vi "NanonisProperties_tessttttt.vi"(0 "Application reference":refnum<vi>, 5 "Ring":u16(ring) items=["all", "setpoint", "zread", "current", "frame", "follow me"], 11 "Error in":errorcluster, 12 "Z Write?":bool) -> (4 "Application ref out":refnum<vi>, 14 "tick count":u32, 15 "error out":errorcluster)   [LabVIEW 2019]
uses:
  <userlib>/Nanonis Prog Interface V5/Nanonis Prog Interface.lvlib
panel:
  out "Z Read (m)":sgl format="%#_6p"
  in  "Z Write (m)":sgl format="%#_6p"
  out "Setpoint (A)":sgl format="%#_6p"
  out "Current (pA)":sgl format="%#_6p"
  in  "Z pen (nm)":dbl
  in  "X pen (nm)":dbl
  out "Frame Size (m)":cluster{"Width":sgl, "Height":sgl} {"Height" format="%.2p"; "Width" format="%.2p"}
  out "Frame Origin (m)":cluster{"Xc":sgl, "Yc":sgl} {"Yc" format="%.2p"; "Xc" format="%.2p"}
  out "prog int?":bool
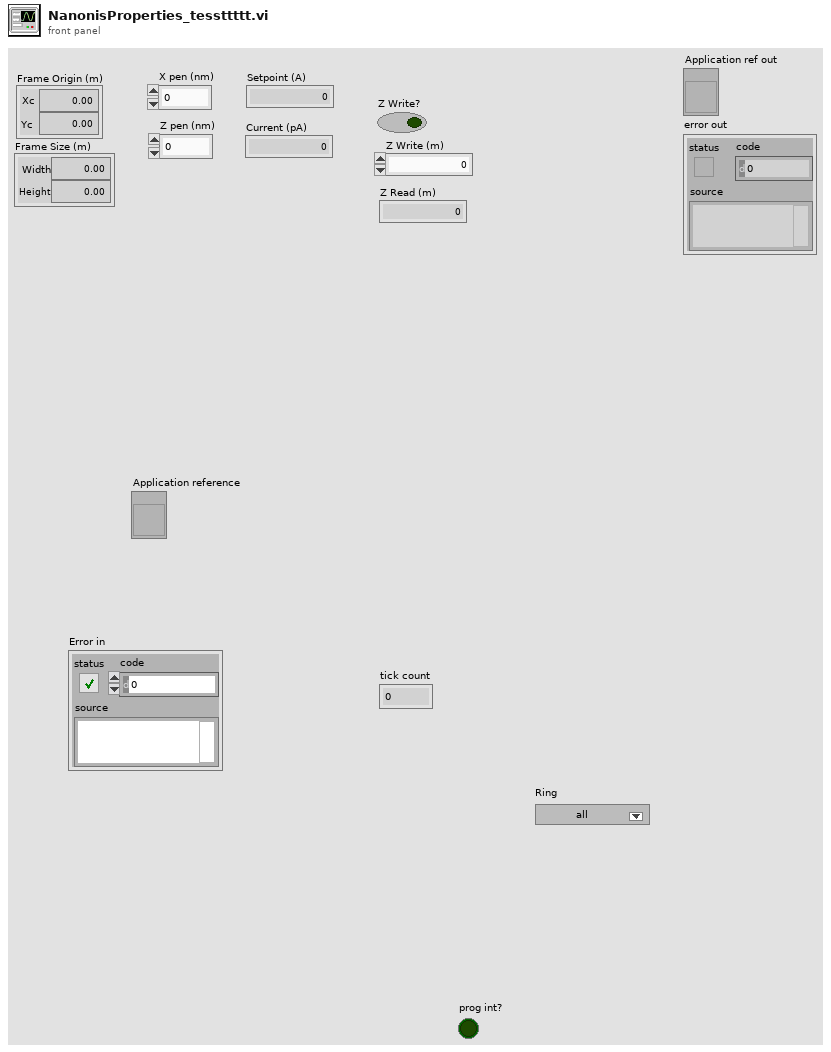
[diagram p1: front panel]
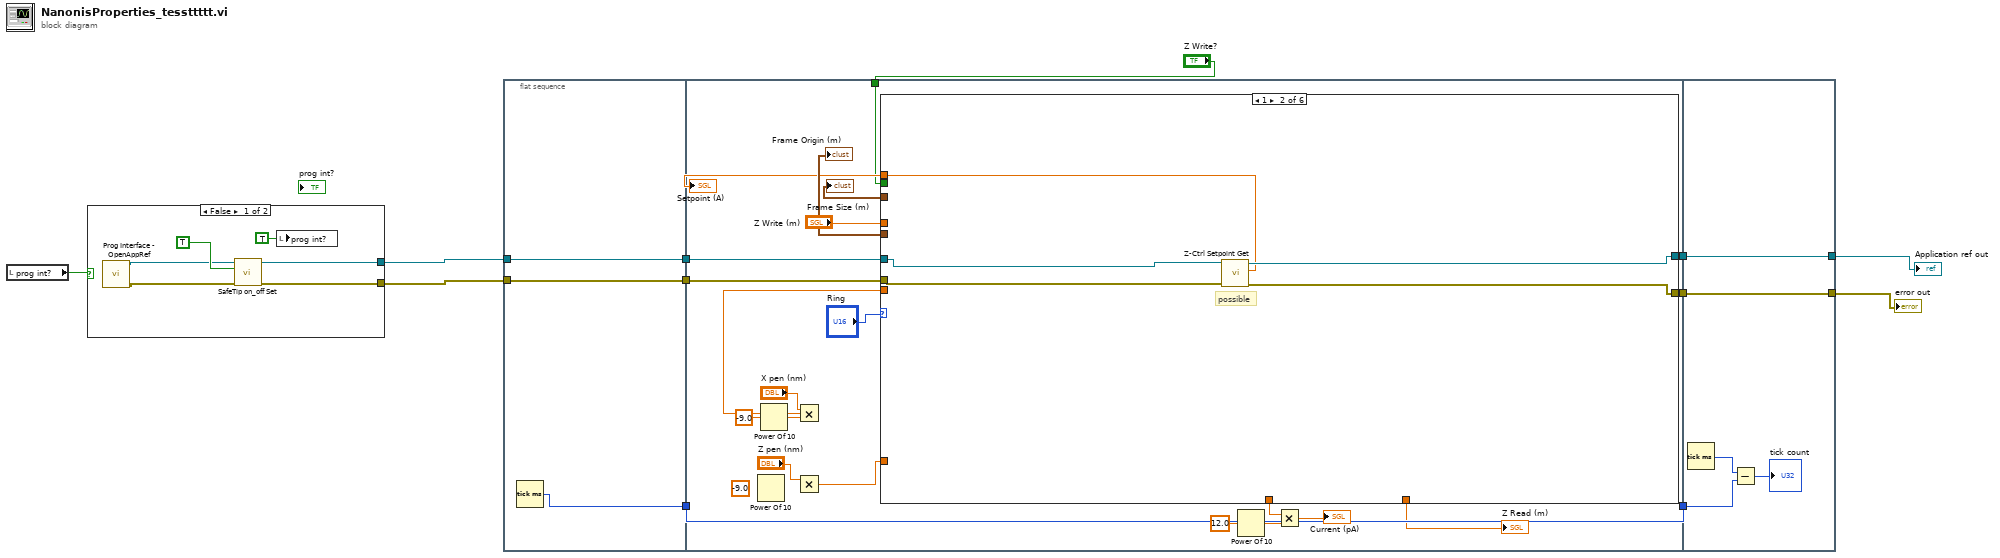
[diagram p0: block diagram]
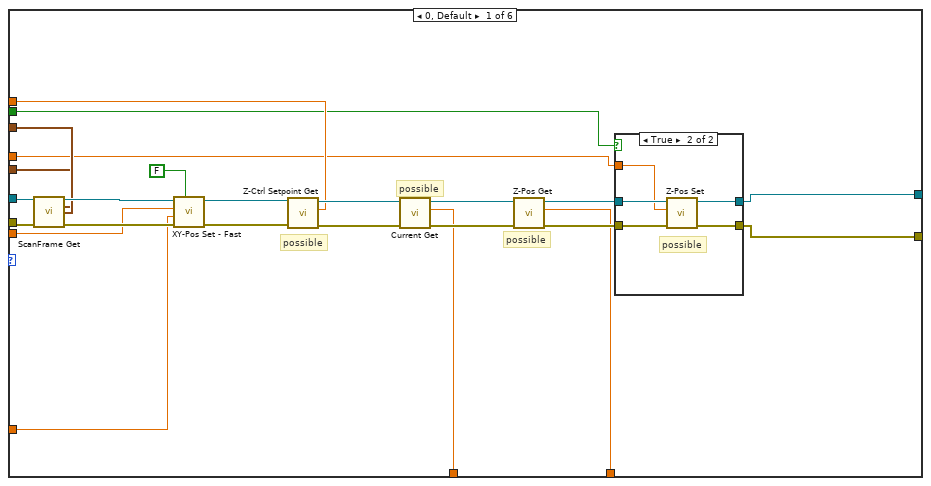
[diagram p2: hidden frame]
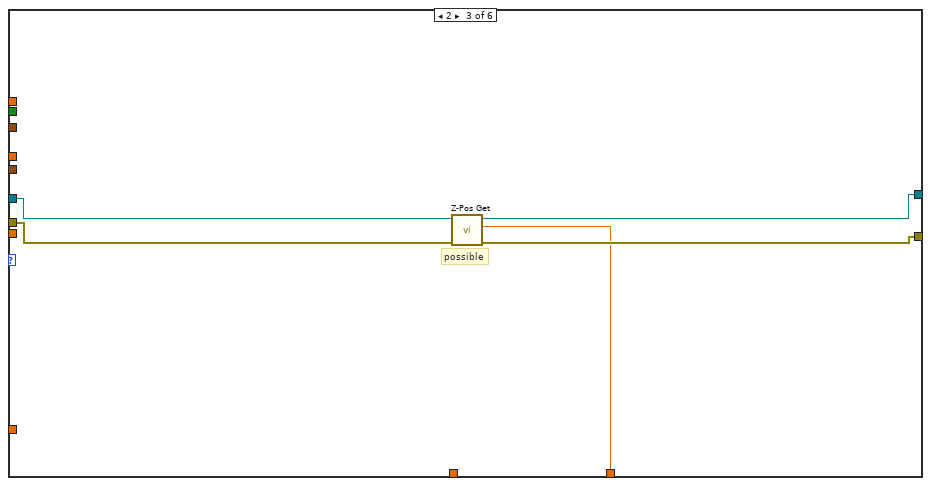
[diagram p4: hidden frame]
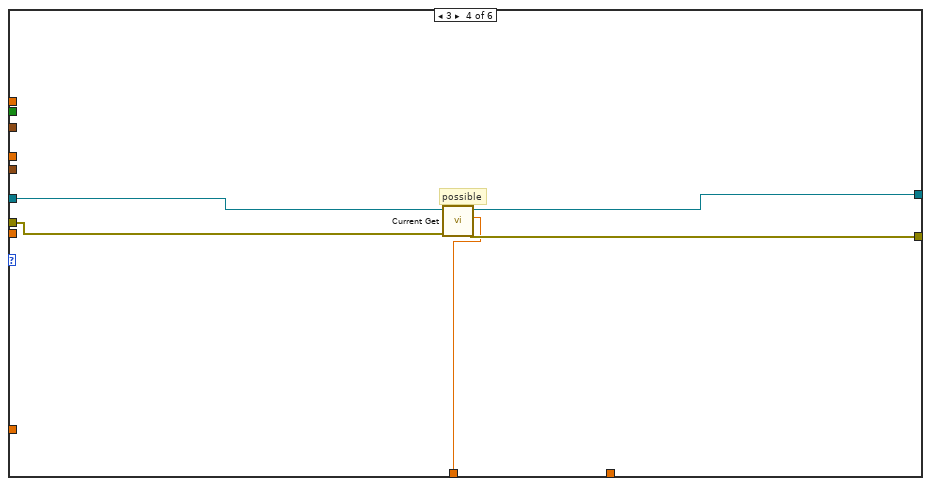
[diagram p5: hidden frame]
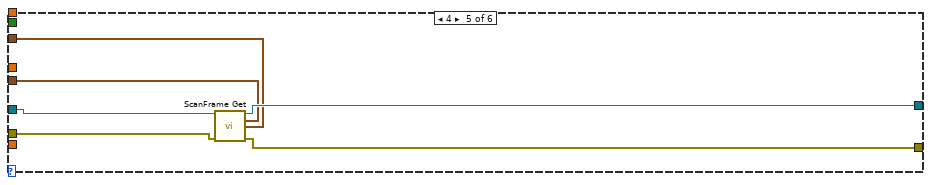
[diagram p6: hidden frame]
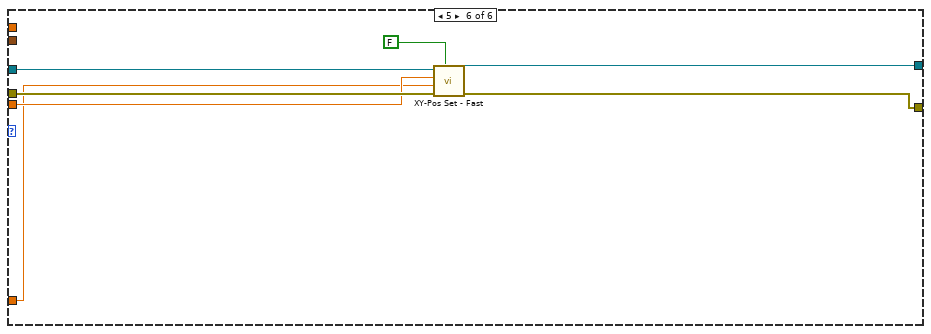
[diagram p7: hidden frame]
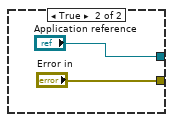
[diagram p8: hidden frame]
diagram:
  n1 = local read "prog int?"() -> (w10:bool)
  n2 = case shown="False" w10 {
    tunnel: [w16 "Application reference"] -> w12
    tunnel: [w15 "Error in"] -> w11
    frame False {
      n3 = call <userlib>:"Prog Interface - OpenAppRef.vi"() -> ("Error out"=w13:errorcluster, "Application reference"=w14:refnum<vi>)  [unwired: 6 in]
      n4 = call <userlib>:"SafeTip on_off Set.vi"("error in (no error)"=w13, "SafeTip ON/OFF"=TRUE, "Application ref in"=w14) -> ("error out"=w15:errorcluster, "Application ref out"=w16:refnum<vi>)  [unwired: 7 in]
      n5 = local write "prog int?"(TRUE ("prog int?")) -> ()
    }
    frame True {
    }
  }
  n6 = flat-sequence {
    tunnel: w11 -> [w22]
    tunnel: w12 -> [w23]
    tunnel: [w23] -> w9
    tunnel: [w22] -> w8
    tunnel: [w21] -> w7
    tunnel: w9 -> [w45]
    tunnel: w8 -> [w44]
    tunnel: w7 -> [w43]
    tunnel: [w43] -> w6
    tunnel: [w41] -> w5
    tunnel: [w40] -> w4
    tunnel: "Z Write?" -> [w30]
    tunnel: w6 -> [w108]
    tunnel: w5 -> [w105]
    tunnel: w4 -> [w106]
    tunnel: [w106] -> w2
    tunnel: [w105] -> w1
    frame #0 {
      n7 = Tick Count (ms)() -> (millisecond timer value=w21:u32)
    }
    frame #1 {
      (unwired) -9.0 ("x")
      n8 = Power Of 10() -> ()  [unwired: 1 in, 1 out]
      n9 = Power Of 10(x=-9.0) -> (10^x=w29:dbl)
      n10 = Multiply(x="X pen (nm)", y=w29) -> (x*y=w24:dbl)
      n11 = Multiply(x="Z pen (nm)") -> (x*y=w25:dbl)  [unwired: 1 in]
      n12 = case shown="1" "Ring" {
        tunnel: w45 -> [w58 w81 w86 w91 w97 w104]
        tunnel: w44 -> [w57 w80 w85 w90 w96 w103]
        tunnel: [w56 w78 w83 w88 w95 w101] -> w41
        tunnel: [w55 w79 w84 w89 w94 w102] -> w40
        tunnel: [w54 _ _ _ w92 _] -> w39
        tunnel: [w53 _ _ _ w93 _] -> w38
        tunnel: w25 -> [w52 _ _ _ _ w98]
        tunnel: w24 -> [w51 _ _ _ _ w99]
        tunnel: [w50 _ _ w87 _ _] -> w34
        tunnel: [w49 _ w82 _ _ _] -> w33
        tunnel: [w48 w77 _ _ _ _] -> w32
        tunnel: "Z Write (m)" -> [w47 _ _ _ _ _]
        tunnel: w30 -> [w46 _ _ _ _ _]
        frame 0, Default {
          # "possible"
          # "possible"
          # "possible"
          n13 = call <userlib>:"ScanFrame Get.vi"("Application ref in"=w58, "error in (no error)"=w57) -> ("Application ref out"=w68:refnum<vi>, "Center coordinates (m)"=w53:cluster{"Xc":sgl, "Yc":sgl}, "Size (m)"=w54:cluster{"Width":sgl, "Height":sgl}, "error out"=w67:errorcluster)  [unwired: 9 in, 1 out]
          n14 = call <userlib>:"XY-Pos Set - Fast.vi"("Wait end-of-motion (T=True)"=FALSE, "error in (no error)"=w67, "Y (m)"=w52, "X (m)"=w51, "Application ref in"=w68) -> ("error out"=w65:errorcluster, "Application ref out"=w66:refnum<vi>)  [unwired: 4 in]
          n15 = call <userlib>:"Z-Ctrl Setpoint Get.vi"("error in (no error)"=w65, "Application ref in"=w66) -> ("error out"=w63:errorcluster, "Z Controller setpoint"=w48:sgl, "Application ref out"=w64:refnum<vi>)  [unwired: 6 in]
          n16 = call <userlib>:"Current Get.vi"("Error in (no error)"=w63, "Application ref in"=w64) -> ("Error out"=w61:errorcluster, "Current (A)"=w50:sgl, "Application ref out"=w62:refnum<vi>)  [unwired: 5 in]
          n17 = call <userlib>:"Z-Pos Get.vi"("error in (no error)"=w61, "Application ref in"=w62) -> ("error out"=w59:errorcluster, "Z position (m)"=w49:sgl, "Application ref out"=w60:refnum<vi>)  [unwired: 7 in]
          n18 = case shown="True" w46 {
            tunnel: w60 -> [w71 w76]
            tunnel: w59 -> [w70 w75]
            tunnel: [w71 w74] -> w55
            tunnel: [w70 w73] -> w56
            tunnel: w47 -> [_ w72]
            frame False {
            }
            frame True {
              # "possible"
              n19 = call <userlib>:"Z-Pos Set.vi"("error in (no error)"=w75, "Z position (m)"=w72, "Application ref in"=w76) -> ("error out"=w73:errorcluster, "Application ref out"=w74:refnum<vi>)  [unwired: 7 in]
            }
          }
        }
        frame 1 {
          # "possible"
          n20 = call <userlib>:"Z-Ctrl Setpoint Get.vi"("error in (no error)"=w80, "Application ref in"=w81) -> ("error out"=w78:errorcluster, "Z Controller setpoint"=w77:sgl, "Application ref out"=w79:refnum<vi>)  [unwired: 6 in]
        }
        frame 2 {
          # "possible"
          n21 = call <userlib>:"Z-Pos Get.vi"("error in (no error)"=w85, "Application ref in"=w86) -> ("error out"=w83:errorcluster, "Z position (m)"=w82:sgl, "Application ref out"=w84:refnum<vi>)  [unwired: 7 in]
        }
        frame 3 {
          # "possible"
          n22 = call <userlib>:"Current Get.vi"("Error in (no error)"=w90, "Application ref in"=w91) -> ("Error out"=w88:errorcluster, "Current (A)"=w87:sgl, "Application ref out"=w89:refnum<vi>)  [unwired: 5 in]
        }
        frame 4 {
          n23 = call <userlib>:"ScanFrame Get.vi"("Application ref in"=w97, "error in (no error)"=w96) -> ("Application ref out"=w94:refnum<vi>, "Center coordinates (m)"=w93:cluster{"Xc":sgl, "Yc":sgl}, "Size (m)"=w92:cluster{"Width":sgl, "Height":sgl}, "error out"=w95:errorcluster)  [unwired: 9 in, 1 out]
        }
        frame 5 {
          n24 = call <userlib>:"XY-Pos Set - Fast.vi"("Wait end-of-motion (T=True)"=FALSE, "error in (no error)"=w103, "Y (m)"=w98, "X (m)"=w99, "Application ref in"=w104) -> ("error out"=w101:errorcluster, "Application ref out"=w102:refnum<vi>)  [unwired: 4 in]
        }
      }
      "Frame Origin (m)" <- w38
      "Frame Size (m)" <- w39
      "Z Read (m)" <- w33
      "Setpoint (A)" <- w32
      n25 = Power Of 10(x=12.0) -> (10^x=w37:dbl)
      n26 = Multiply(x=w34, y=w37) -> (x*y=→"Current (pA)":dbl)
    }
    frame #2 {
      n27 = Tick Count (ms)() -> (millisecond timer value=w109:u32)
      n28 = Subtract(x=w109, y=w108) -> (x-y=→"tick count":u32)
    }
  }
  "Application ref out" <- w2
  "error out" <- w1
